vi "dfd_Compute Group Delay from Zeros.vi"(10 "roots":cdb[](array[numeric]), 11 "freq points":dbl[](array[numeric])) -> (2 "# zero root":i32, 3 "group delay":dbl[](array[numeric]))   [LabVIEW 2017, in "NI_DigFilterLicensed.lvlib"]
uses:
  <vilib>/addons/Digital Filter Design/NI_DigFilterLicensed.lvlib
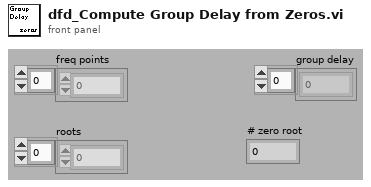
[diagram p1: front panel]
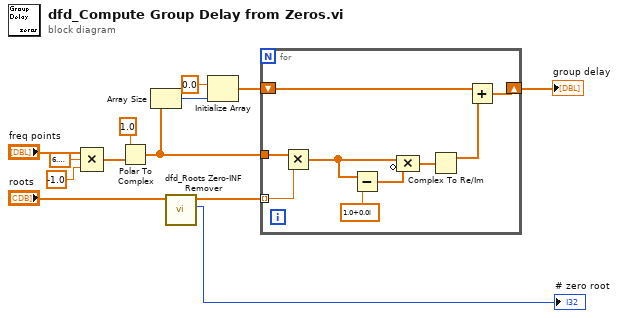
[diagram p0: block diagram]
diagram:
  n1 = Compound Arithmetic op=MULTIPLY("freq points", 6.283185307179586, -1.0 ("value")) -> (w6:dbl[])
  n2 = Polar To Complex(1:w6, 2:1.0) -> (0:w5:cdb[])
  n3 = Array Size(array=w5) -> (size(s)=w12:i32)
  n4 = call <vilib>:"dfd_Roots Zero-INF Remover.vi"("roots"="roots") -> ("# zero root"=→"# zero root":i32, "new roots"=w1:cdb[])  [unwired: 9 out]
  n5 = Initialize Array(0.0, w12) -> (w13:dbl[])
  n6 = for {
    tunnel: w5 -> [w16]
    shift-right: [w21] -> w10
    shift-left: w13 -> [w22]
    tunnel: w1 -> [w15] mode=indexing
    n7 = Multiply(x=w16, y=w15) -> (x*y=w18:cdb[])
    n8 = Subtract(x=w18, y=cdb 1.0+0.0i ("x")) -> (x-y=w19:cdb[])
    n9 = Compound Arithmetic op=MULTIPLY(w18, invert w19) -> (w20:cdb[])
    n10 = Complex To Re/Im(x + iy=w20) -> (x=w14:dbl[])  [unwired: 1 out]
    n11 = Add(x=w22, y=w14) -> (x+y=w21:dbl[])
  }
  "group delay" <- w10
